vi "Enter Remote Mode.vi"(8 "error in (no error)":errorcluster, 11 "ASIA Pump #":i32) -> (0 "error out":errorcluster, 2 "Completed":bool=TRUE, 3 "ASIA Pump #":i32)   [LabVIEW 2018, in "ASIA Pump.lvlib"]
uses:
  ASIA Pump.lvlib
panel:
  out "path out":path
  out "error out 2":errorcluster
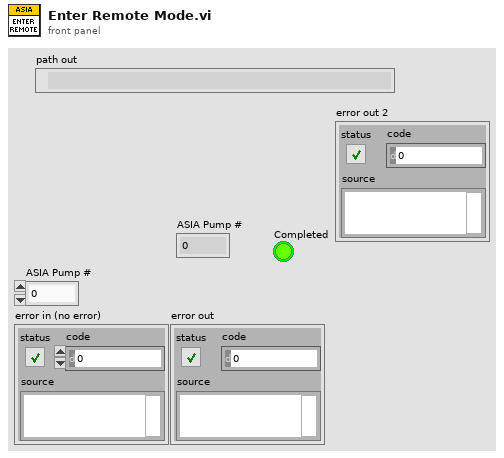
[diagram p1: front panel]
types:
  T1 = cluster{"Busy":bool, "PumpCnt":dbl, "RemoteEntered":bool, "OverpressureSet":bool}[]
  T2 = cluster{"Busy":bool, "PumpCnt":dbl, "RemoteEntered":bool, "OverpressureSet":bool}
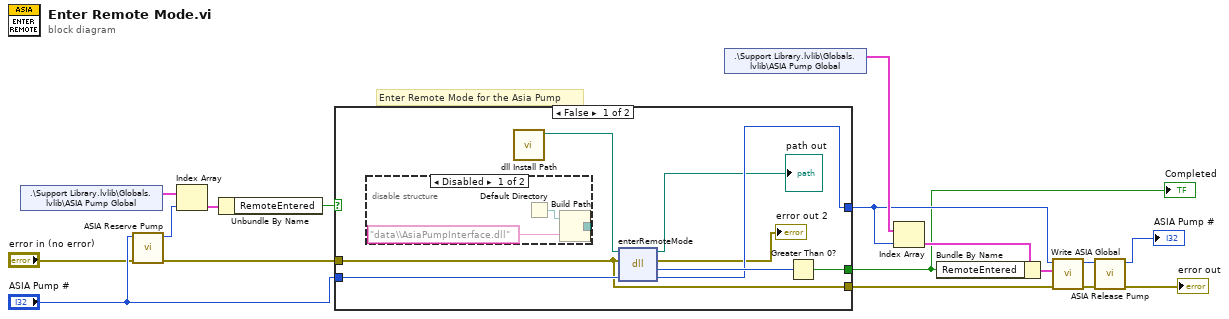
[diagram p0: block diagram]
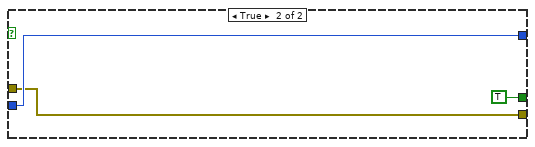
[diagram p3: hidden frame]
diagram:
  # "Enter Remote Mode for the Asia Pump"
  n1 = shared-variable ".\\Support Library.lvlib\\Globals.lvlib\\ASIA Pump Global"() -> (w17:T1)  [unwired: 1 in, 1 out]
  n2 = call "ASIA Reserve Pump.vi"("error in (no error)"="error in (no error)", "ASIA Pump # In"="ASIA Pump #") -> ("error out"=w11:errorcluster, "ASIA Pump # Out"=w13:i32)  [unwired: 8 in]
  n3 = Index Array(array=w17, index=w13) -> (element=w16:T2)
  n4 = Unbundle By Name(w16) -> ("RemoteEntered"=w15:bool)
  n5 = case shown="False" w15 {
    tunnel: w11 -> [w21 w29]
    tunnel: "ASIA Pump #" -> [w25 w30]
    tunnel: [w23 TRUE] -> w5
    tunnel: [w22 w30] -> w6
    tunnel: [w21 w29] -> w7
    frame False {
      n6 = disable-structure shown="Disabled" {
        disable-tunnel: [w26 _] -> _
        frame Disabled {
          n7 = Default Directory() -> (w27:path)
          n8 = Build Path(base path=w27, name or relative path="data\\AsiaPumpInterface.dll") -> (appended path=w26:path)
        }
        frame Enabled {
        }
      }
      n9 = call "dll Install Path.vi"() -> ("system directory"=w19:path)  [unwired: 11 in]
      n10 = dll-call lib="C:/Program Files (x86)/Pfizer/FAST/data/AsiaPumpInterface.dll" fn="enterRemoteMode"(path in=w19, error in=w21, "pumpNum"=w25) -> (path out=→"path out":path, error out=→"error out 2":errorcluster, "return type"=w24:i8, "pumpNum"=w22:u32)  [unwired: 1 in]
      n11 = Greater Than 0?(x=w24) -> (x > 0?=w23:bool)
    }
    frame True {
    }
  }
  "Completed" <- w5
  n12 = shared-variable ".\\Support Library.lvlib\\Globals.lvlib\\ASIA Pump Global"() -> (w9:T1)  [unwired: 1 in, 1 out]
  n13 = Index Array(array=w9, index=w6) -> (element=w10:T2)
  n14 = Bundle By Name(cluster=w10, "RemoteEntered"=w5) -> (w8:T2)
  n15 = call "Write ASIA Global.vi"("error in (no error)"=w7, "ASIA Global"=w8, "Pump Number In"=w6) -> ("error out"=w3:errorcluster, "Pump Number Out"=w4:i32)  [unwired: 7 in]
  n16 = call "ASIA Release Pump.vi"("error in (no error)"=w3, "pumpNum"=w4) -> ("error out"=→"error out":errorcluster, "ASIA Pump # Out"=→"ASIA Pump #":i32)  [unwired: 8 in]
